vi "readSettings.vi"(8 "error in (no error)":errorcluster, 11 "Settings in":refnum<class "Settings.lvclass">) -> (0 "error out":errorcluster, 3 "Settings out":refnum<class "Settings.lvclass">)   [LabVIEW 2016, in "Settings.lvclass"]
uses:
  Settings.lvclass
  Settings.lvclass/Settings.ctl
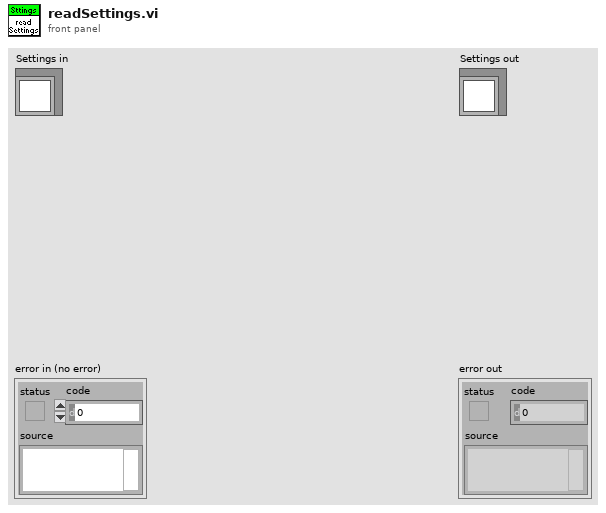
[diagram p1: front panel]
types:
  T1 = enum16{"open", "replace", "create", "open or create", "replace or create", "replace or create with confirmation"}
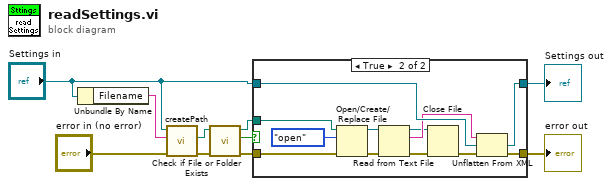
[diagram p0: block diagram]
diagram:
  n1 = Unbundle By Name("Settings in") -> ("Filename"=w10:string)
  n2 = call "createPath.vi"("error in (no error)"="error in (no error)", "filename"=w10, "Settings in"="Settings in") -> ("error out"=w3:errorcluster, "Path"=w5:path)  [unwired: 6 in, 1 out]
  n3 = call <vilib>:"Check if File or Folder Exists.vi"("error in (no error)"=w3, "path"=w5) -> ("error out"=w2:errorcluster, "file or folder exists?"=w4:bool, "dup path"=w1:path)  [unwired: 7 in]
  n4 = case shown="True" w4 {
    tunnel: w2 -> [w11 w24]
    tunnel: w1 -> [_ w22]
    tunnel: "Settings in" -> [w12 w20]
    tunnel: [w12 w19] -> w7
    tunnel: [w11 w18] -> w6
    frame False {
    }
    frame True {
      n5 = Open/Create/Replace File(file path (use dialog)=w22, error in=w24, operation (0:open)=T1."open") -> (refnum out=w14:refnum<file>, error out=w17:errorcluster)  [unwired: 3 in, 1 out]
      n6 = Read from Text File(file (use dialog)=w14, error in=w17) -> (refnum out=w13:refnum<file>, text=w15:string, error out=w16:errorcluster)  [unwired: 2 in, 1 out]
      n7 = Close File(refnum=w13, error in=w16) -> (error out=w21:errorcluster)  [unwired: 1 out]
      n8 = Unflatten From XML(xml string=w15, type=w20, error in (no error)=w21) -> (value=w19:refnum<class "Settings.lvclass">, error out=w18:errorcluster)
    }
  }
  "error out" <- w6
  "Settings out" <- w7
